vi "Main_Acquisition.vi"(8 "error in":errorcluster, 11 "Queues in":T1) -> (0 "error out":errorcluster, 3 "Stop?":bool)   [LabVIEW 2019]
uses:
  Queue/TypeDef/#TypeDef_MyRIO_Queues.ctl
  Data Processing/TypeDef/#TypeDef_PropFromDAtoDP.ctl
  Communication/TypeDef/#TypeDef_FromPCtoMR.ctl
  Communication/TypeDef/#TypeDef_Command.ctl
  Communication/TypeDef/#TypeDef_ErrorHandler_prop.ctl
  Communication/TypeDef/#TypeDef_FromMRtoPC.ctl
  Communication/TypeDef/#TypeDef_PropGraph.ctl
  Communication/TypeDef/#TypeDef_PropertiesToSave.ctl
  TypeDef/#TypeDef_EnumOp_DataAcquisition.ctl
  Communication/TypeDef/#TypeDef_SetGet.ctl
  <vilib>/Platform/TimedLoop/XDataNode/timing_clust.ctl
  <vilib>/Platform/TimedLoop/XDataNode/nitl_modes.ctl
  <vilib>/Platform/TimedLoop/XDataNode/wakeup.ctl
  <vilib>/platform/TimedLoop/XDataNode/XDataNode.xnode
  <vilib>/Platform/TimedLoop/XDataNode/XDNodeRunTimeDep.lvlib
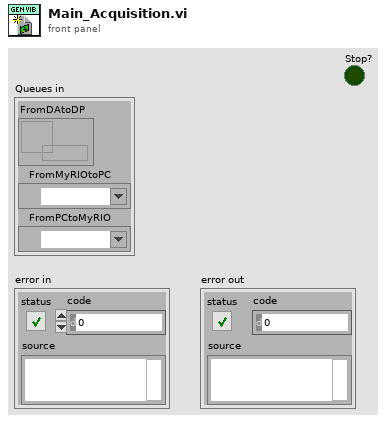
[diagram p1: front panel]
types:
  T1 = typedef "#TypeDef_MyRIO_Queues.ctl" = cluster{"FromDAtoDP":refnum<queue>, "FromMyRIOtoPC":refnum<k21>, "FromPCtoMyRIO":refnum<k21>}
  T2 = typedef "#TypeDef_SetGet.ctl" = enum16{"Set", "Get"}
  T3 = typedef "#TypeDef_FromPCtoMR.ctl" = cluster{"Command":T4, "Error?":bool, "Stop":bool, "StopPomiar":bool, "Name":string, "FilesPath":path, "ErrorHandler":T5, "Fs":dbl}
  T4 = typedef "#TypeDef_Command.ctl" = enum16{"Start", "End"}
  T5 = typedef "#TypeDef_ErrorHandler_prop.ctl" = cluster{"Threads":enum16{"Acquisistion", "Data Operation", "Save File"}, "ClearError":bool, "Error Out ":errorcluster, "Error":bool}
  T6 = typedef "#TypeDef_EnumOp_DataAcquisition.ctl" = enum16{"Idle", "Init", "Acq", "End", "Error_Shutdown", "ClearError"}
  T7 = typedef "#TypeDef_PropFromDAtoDP.ctl" = cluster{"Accessibility":T3, "RawData":dbl[][], "Counter":i32, "Fs":dbl}
  T8 = typedef "XDNodeRunTimeDep.lvlib/timing_clust.ctl" = cluster{"Expected End [f-1]":u64, "Actual End [f-1]":u64, "Finished Late? [f-1]":bool, "Expected End [i-1]":u64, "Actual End [i-1]":u64, "Finished Late? [i-1]":bool, "Expected Start [i]":u64, "Actual Start [i]":u64, "Expected Start [f]":u64, "Actual Start [f]":u64, "Source Name":string, "Structure Name":string, "Period":i64, "Deadline":i64, "Offset":i64, "Start":i64, "Priority":i32, "Timeout":i32, "Mode":T9, "Wakeup Reason":T10, "Error":errorcluster, "Source Type":string, "Secondary Source Type":string, "Global End Time":u64, "Global Start Time":u64, "Frame Duration":u64, "Iteration Duration":u64, "Assigned CPU":i32, "I/O Scan Engine Mode":u32}
  T9 = typedef "XDNodeRunTimeDep.lvlib/nitl_modes.ctl" = enum32{"No Change", "Process missed periods, maintain original phase", "Discard missed periods, maintain original phase", "Process missed periods, ignore original phase", "Discard missed periods, ignore original phase"}
  T10 = typedef "XDNodeRunTimeDep.lvlib/wakeup.ctl" = enum32{"Normal", "Aborted", "Asynchronous wakeup", "Timing source error", "Timed loop error", "Timeout"}
  T11 = typedef "AI.lvlib/AI Reference.ctl" = cluster{"myRIO Reference":T12, "AI Channels List":T16, "AI Scaling Constants List":T18}
  T12 = typedef "myRIO Generic Hardware Reference.ctl" = cluster{"myRIO Model":T13, "myRIO Hardware Reference":T14}
  T13 = typedef "Hardware Version Enum.ctl" = enum16{"Unknown", "myRIO-1900", "myRIO-1950", "roboRIO", "NI ELVIS RIO CM", "ELVIS III"}
  T14 = typedef "myRIO v1.0 Reference.ctl" = cluster{"Generic FPGA Reference":T15, "Allow multiple opens":bool}
  T15 = typedef "Generic FPGA Reference.ctl" = refnum<k20>
  T16 = typedef "AI Channels List.ctl" = T17[]
  T17 = typedef "AI Channels Enum.ctl" = enum16{"Not Connected", "AudioIn/Left", "AudioIn/Right", "C/AI0", "C/AI1", "A/AI0", "A/AI1", "A/AI2", "A/AI3", "A/AI4", "A/AI5", "A/AI6", "A/AI7", "B/AI0", "B/AI1", "B/AI2", "B/AI3", "B/AI4", "B/AI5", "B/AI6", "B/AI7", "AI/AI0", "AI/AI1", "AI/AI2", "AI/AI3", "A/AI0 (DIFF)", "A/AI1 (DIFF)", "A/AI2 (DIFF)", "A/AI3 (DIFF)", "B/AI0 (DIFF)", "B/AI1 (DIFF)", "B/AI2 (DIFF)", "B/AI3 (DIFF)"}
  T18 = typedef "Analog Scaling Constants List.ctl" = T19[]
  T19 = typedef "Analog Scaling Constants.ctl" = cluster{"LSB Weight (Volts)":dbl, "Offset (Volts)":dbl, "Signed?":bool}
  T20 = typedef "I2C.lvlib/I2C Reference.ctl" = cluster{"myRIO Reference":T12, "I2C Channels Enum":T21, "I2C Configuration":T22}
  T21 = typedef "I2C Channels Enum.ctl" = enum16{"Not Connected", "A/I2C", "B/I2C", "I2C/I2C"}
  T22 = typedef "I2C.lvlib/I2C Configuration.ctl" = cluster{"I2C Transfer Rate":T23}
  T23 = typedef "I2C.lvlib/I2C Transfer Rate.ctl" = enum16{"Standard mode (100 kbps)", "Fast mode (400 kbps)"}
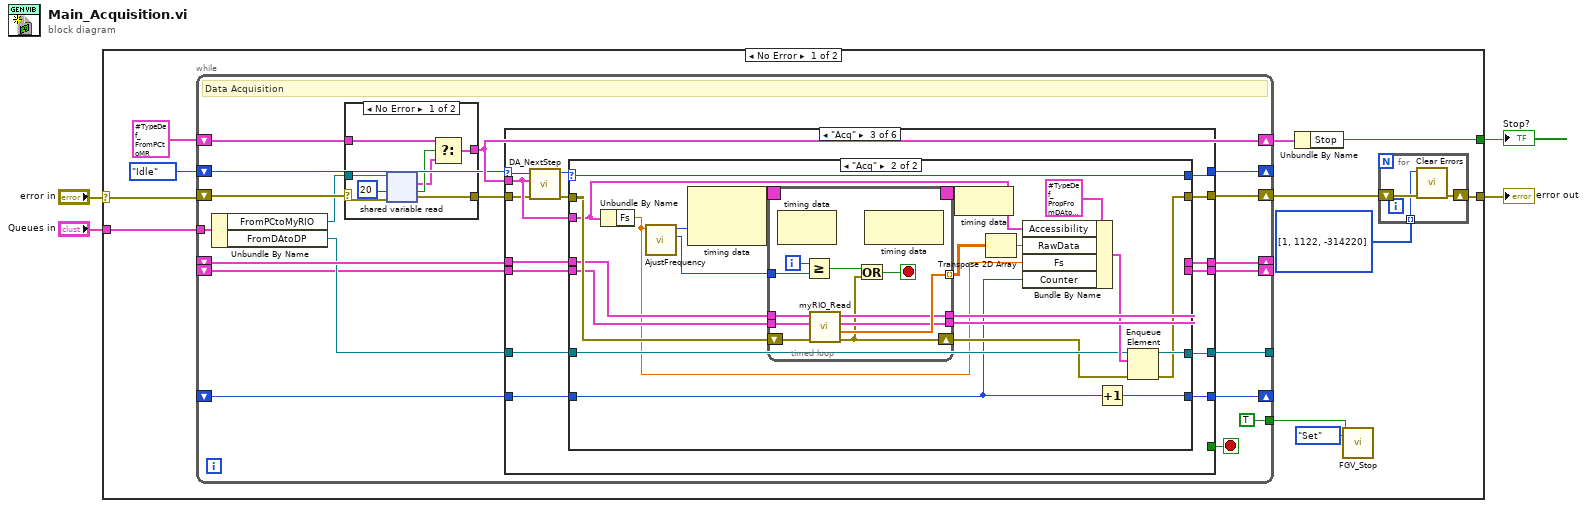
[diagram p0: block diagram]
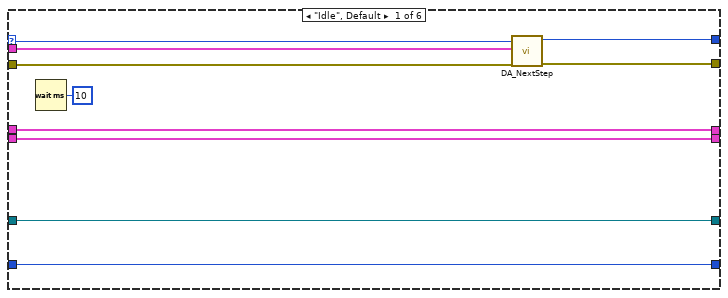
[diagram p3: hidden frame]
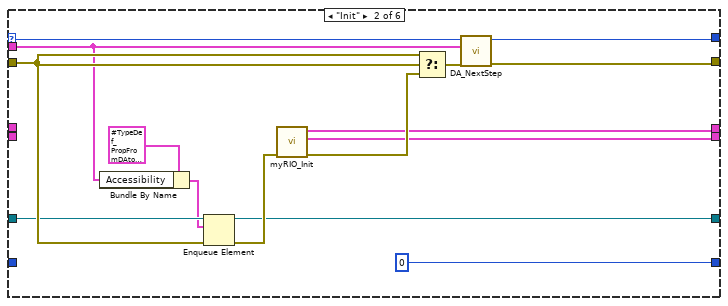
[diagram p4: hidden frame]
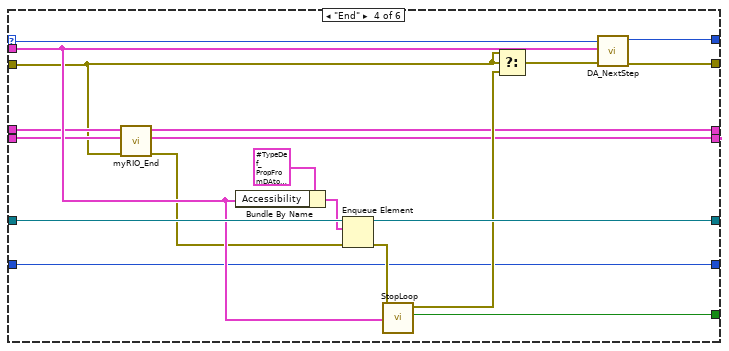
[diagram p6: hidden frame]
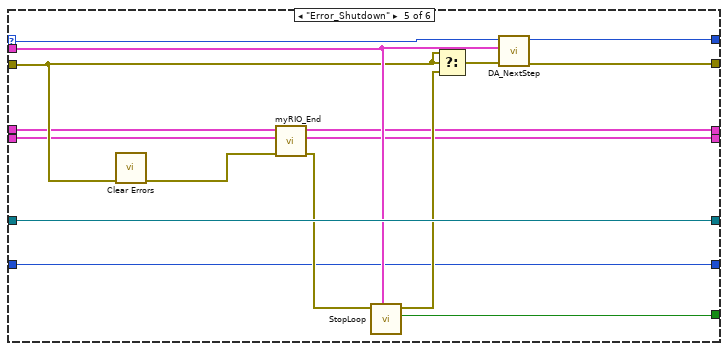
[diagram p7: hidden frame]
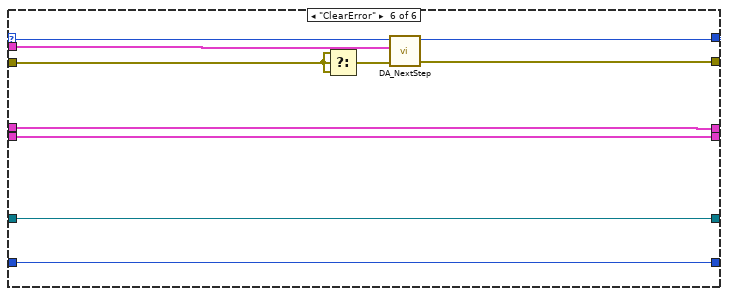
[diagram p8: hidden frame]
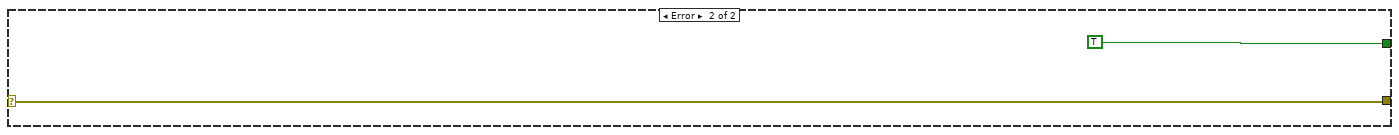
[diagram p9: hidden frame]
diagram:
  n1 = case shown="No Error" "error in" {
    selector: "error in" -> [w15 w179]
    tunnel: "Queues in" -> [w14 _]
    tunnel: [w8 w179] -> w3
    tunnel: [w10 TRUE ("Stop")] -> w1
    frame No Error {
      n2 = while {
        shift-right: [w32] -> _
        shift-left: #TypeDef_EnumOp_DataAcquisition."Idle" ("EnumOp_DataAcquisition") -> [w26]
        tunnel: w14 -> [w31]
        shift-right: [w35] -> _
        shift-left: _ -> [w34]
        shift-right: [w33] -> w9
        shift-left: w15 -> [w37]
        tunnel: [w28] -> _
        shift-right: [w27] -> w11
        shift-left: T3 {"Command"=enum."End", "Error?"=FALSE, "Stop"=FALSE, "StopPomiar"=FALSE, "Name"="", "FilesPath"=path "", "ErrorHandler"={"Threads"=enum."Acquisistion", "ClearError"=FALSE, "Error Out "={"status"=FALSE, "code"=0, "source"=""}, "Error"=FALSE}, "Fs"=0.0} ("PCtoMyRio") -> [w36]
        shift-right: [w24] -> _
        shift-left: _ -> [w23]
        shift-right: [w22] -> _
        shift-left: _ -> [w21]
        tunnel: [TRUE ("STOP in")] -> w5
        stop <- w20 stop-if-true
        # "Data Acquisition"
        n3 = Unbundle By Name(w31) -> ("FromPCtoMyRIO"=w30:refnum<k21>, "FromDAtoDP"=w29:refnum<queue>)
        n4 = case shown="No Error" w37 {
          selector: w37 -> [w43 w47]
          tunnel: [w38 w47] -> w25
          tunnel: [w44 w46] -> w27
          tunnel: w36 -> [w45 w46]
          tunnel: w30 -> [w42 _]
          frame No Error {
            n5 = shared-variable-read(w42, w43, 20 ("timeout in ms (-1)")) -> (w38:errorcluster, w40:bool, w39:T3)  [unwired: 1 out]
            n6 = Select(t=w45, s=w40, f=w39) -> (s? t:f=w44:T3)
          }
          frame Error {
          }
        }
        n7 = case shown="\"Acq\"" w26 {
          selector: w26 -> [w55 w70 w87 w148 w166 w172]
          tunnel: w27 -> [w51 w58 w82 w141 w161 w173]
          tunnel: w25 -> [w56 w63 w81 w137 w159 w174]
          tunnel: [w52 w67 w83 w136 w155 w177] -> w35
          tunnel: w34 -> [w52 _ w84 w139 w158 w177]
          tunnel: [w57 w71 w79 w150 w164 w175] -> w33
          tunnel: [w54 w69 w77 w149 w165 w171] -> w32
          tunnel: w29 -> [w48 w62 w86 w147 w163 w170]
          tunnel: [w48 w61 w85 w146 w163 w170] -> w28
          tunnel: [_ _ _ w140 w160 _] -> w20
          tunnel: [w50 w66 w76 w135 w156 w169] -> w24
          tunnel: w23 -> [w50 _ w75 w138 w157 w169]
          tunnel: [w49 0 ("Counter") w74 w133 w152 w168] -> w22
          tunnel: w21 -> [w49 _ w73 w133 w152 w168]
          frame "Idle", Default {
            n8 = Wait (ms)(milliseconds to wait=u32 10) -> ()  [unwired: 1 out]
            n9 = call "DA_NextStep.vi"("error in"=w56, "PCtoMyRio"=w51, "PreviousStep"=w55) -> ("error out"=w57:errorcluster, "NextStep"=w54:T6)  [unwired: 7 in]
          }
          frame "Init" {
            n10 = Bundle By Name(cluster=T7 {"Accessibility"={"Command"=enum."Start", "Error?"=FALSE, "Stop"=FALSE, "StopPomiar"=FALSE, "Name"="", "FilesPath"=path "", "ErrorHandler"={"Threads"=enum."Acquisistion", "ClearError"=FALSE, "Error Out "={"status"=FALSE, "code"=0, "source"=""}, "Error"=FALSE}, "Fs"=0.0}, "RawData"=[], "Counter"=0, "Fs"=0.0}, "Accessibility"=w58) -> (w59:T7)
            n11 = Enqueue Element(queue=w62, element=w59, error in (no error)=w63) -> (queue out=w61:refnum<queue>, error out=w64:errorcluster)  [unwired: 1 in, 1 out]
            n12 = call "myRIO_Init.vi"("error in"=w64) -> ("error out"=w68:errorcluster, "AI Ref Out"=w66:T11, "I2C Ref Out"=w67:T20)  [unwired: 8 in]
            n13 = Select(t=w63, s=w63, f=w68) -> (s? t:f=w72:errorcluster)
            n14 = call "DA_NextStep.vi"("error in"=w72, "PCtoMyRio"=w58, "PreviousStep"=w70) -> ("error out"=w71:errorcluster, "NextStep"=w69:T6)  [unwired: 7 in]
          }
          frame "Acq" {
            n15 = call "DA_NextStep.vi"("error in"=w81, "PCtoMyRio"=w82, "PreviousStep"=w87) -> ("error out"=w80:errorcluster, "NextStep"=w78:T6)  [unwired: 7 in]
            n16 = case shown="\"Acq\"" w78 {
              selector: w78 -> [w90 w115]
              tunnel: w86 -> [w91 w103]
              tunnel: [w91 w105] -> w85
              tunnel: w84 -> [w92 w113]
              tunnel: [w92 w107] -> w83
              tunnel: w82 -> [_ w95]
              tunnel: w80 -> [w93 w114]
              tunnel: [w93 w101] -> w79
              tunnel: [w90 w115] -> w77
              tunnel: [w89 w106] -> w76
              tunnel: w75 -> [w89 w112]
              tunnel: [w88 w98] -> w74
              tunnel: w73 -> [w88 w97]
              frame "End", Default {
              }
              frame "Acq" {
                n17 = Unbundle By Name(w95) -> ("Fs"=w94:dbl)
                n18 = call "AjustFrequency.vi"("Frequency"=w94) -> ("N elements"=w109:i32, "dt"=w100:i64)  [unwired: 9 in]
                n19 = node-c288(w100) -> (w111:T8)  [unwired: 1 in]
                n20 = timed-loop "Timed Loop" {
                  timing: w111 -> [_]
                  timing-out: [_] -> w110
                  tunnel: w113 -> [w125]
                  tunnel: w112 -> [w124]
                  shift-right: [w116] -> w102
                  shift-left: w114 -> [w126]
                  tunnel: w109 -> [w122]
                  tunnel: [w120] -> w96 mode=indexing
                  tunnel: [w119] -> w107
                  tunnel: [w118] -> w106
                  i -> [w123]
                  stop <- w121 stop-if-true
                  n21 = node-c288() -> ()  [unwired: 1 in, 1 out]
                  n22 = Greater Or Equal?(x=w123, y=w122) -> (x >= y?=w117:bool)
                  n23 = call "myRIO_Read.vi"("error in"=w126, "AI Ref In"=w124, "I2C Ref Out in"=w125) -> ("error out"=w116:errorcluster, "Data"=w120:dbl[], "AI Ref Out"=w118:T11, "I2C Ref Out out"=w119:T20)  [unwired: 5 in]
                  n24 = Or(x=w117, y=w116) -> (x .or. y?=w121:bool)
                  n25 = node-c288() -> ()  [unwired: 1 in, 1 out]
                }
                n26 = node-c288(w110) -> ()
                n27 = Transpose 2D Array(2D array=w96) -> (transposed array=w99:dbl[][])
                n28 = Bundle By Name(cluster=T7 {"Accessibility"={"Command"=enum."Start", "Error?"=FALSE, "Stop"=FALSE, "StopPomiar"=FALSE, "Name"="", "FilesPath"=path "", "ErrorHandler"={"Threads"=enum."Acquisistion", "ClearError"=FALSE, "Error Out "={"status"=FALSE, "code"=0, "source"=""}, "Error"=FALSE}, "Fs"=0.0}, "RawData"=[], "Counter"=0, "Fs"=0.0}, "Accessibility"=w95, "RawData"=w99, "Fs"=w94, "Counter"=w97) -> (w104:T7)
                n29 = Increment(x=w97) -> (x+1=w98:i32)
                n30 = Enqueue Element(queue=w103, element=w104, error in (no error)=w102) -> (queue out=w105:refnum<queue>, error out=w101:errorcluster)  [unwired: 1 in, 1 out]
              }
            }
          }
          frame "End" {
            n31 = call "myRIO_End.vi"("error in (no error)"=w137, "AI Ref in"=w138, "I2C Ref in"=w139) -> ("error out"=w134:errorcluster, "AI Ref out"=w135:T11, "I2C Ref Out"=w136:T20)  [unwired: 6 in]
            n32 = Bundle By Name(cluster=T7 {"Accessibility"={"Command"=enum."Start", "Error?"=FALSE, "Stop"=FALSE, "StopPomiar"=FALSE, "Name"="", "FilesPath"=path "", "ErrorHandler"={"Threads"=enum."Acquisistion", "ClearError"=FALSE, "Error Out "={"status"=FALSE, "code"=0, "source"=""}, "Error"=FALSE}, "Fs"=0.0}, "RawData"=[], "Counter"=0, "Fs"=0.0}, "Accessibility"=w141) -> (w144:T7)
            n33 = Enqueue Element(queue=w147, element=w144, error in (no error)=w134) -> (queue out=w146:refnum<queue>, error out=w143:errorcluster)  [unwired: 1 in, 1 out]
            n34 = call "StopLoop.vi"("Accessibility"=w141, "error in (no error)"=w143) -> ("Stop?"=w140:bool, "error out"=w142:errorcluster)  [unwired: 8 in]
            n35 = Select(t=w137, s=w137, f=w142) -> (s? t:f=w151:errorcluster)
            n36 = call "DA_NextStep.vi"("error in"=w151, "PCtoMyRio"=w141, "PreviousStep"=w148) -> ("error out"=w150:errorcluster, "NextStep"=w149:T6)  [unwired: 7 in]
          }
          frame "Error_Shutdown" {
            n37 = call <vilib>:"Clear Errors.vi"("error in (no error)"=w159) -> ("error out"=w154:errorcluster)  [unwired: 5 in, 1 out]
            n38 = call "myRIO_End.vi"("error in (no error)"=w154, "AI Ref in"=w157, "I2C Ref in"=w158) -> ("error out"=w153:errorcluster, "AI Ref out"=w156:T11, "I2C Ref Out"=w155:T20)  [unwired: 6 in]
            n39 = call "StopLoop.vi"("Accessibility"=w161, "error in (no error)"=w153) -> ("Stop?"=w160:bool, "error out"=w162:errorcluster)  [unwired: 8 in]
            n40 = Select(t=w159, s=w159, f=w162) -> (s? t:f=w167:errorcluster)
            n41 = call "DA_NextStep.vi"("error in"=w167, "PCtoMyRio"=w161, "PreviousStep"=w166) -> ("error out"=w164:errorcluster, "NextStep"=w165:T6)  [unwired: 7 in]
          }
          frame "ClearError" {
            n42 = Select(t=w174, s=w174, f=w174) -> (s? t:f=w176:errorcluster)
            n43 = call "DA_NextStep.vi"("error in"=w176, "PCtoMyRio"=w173, "PreviousStep"=w172) -> ("error out"=w175:errorcluster, "NextStep"=w171:T6)  [unwired: 7 in]
          }
        }
      }
      n44 = Unbundle By Name(w11) -> ("Stop"=w10:bool)
      n45 = call "FGV_Stop.vi"("Get/Set"=#TypeDef_SetGet."Set", "STOP in"=w5) -> ()  [unwired: 9 in, 1 out]
      n46 = for {
        shift-right: [w17] -> w8
        shift-left: w9 -> [w18]
        tunnel: i32[] [1, 1122, -314220] -> [w16] mode=indexing
        n47 = call <vilib>:"Clear Errors.vi"("error in (no error)"=w18, "specific error code to clear (0: all)"=w16) -> ("error out"=w17:errorcluster)  [unwired: 4 in, 1 out]
      }
    }
    frame Error {
    }
  }
  "error out" <- w3
  "Stop?" <- w1
